vi "calculator.vi"() -> ()   [LabVIEW 2019]
doc: "Use this template to build a producer/consumer design pattern with events to produce queue items. Use this design pattern instead of the User Interface Event Handler pattern for user interfaces when you want to execute code asynchronously in response to an event without slowing the user interface responsiveness."
uses:
  control/command control.ctl
panel:
  in  "Divide":bool
  in  "Multiply":bool
  out "Array 2":string[](array[string])
  out "Array":dbl[](array[numeric])
  in  "Minus":bool
  in  "Equal":bool
  in  "Add":bool
  in  "Off":bool
  out "error out":errorcluster
  in  "Decimal Point":bool
  in  "Button 9":bool
  in  "Button 8":bool
  in  "Button 7":bool
  in  "Button 6":bool
  in  "Button 5":bool
  in  "Button 4":bool
  in  "Button 3":bool
  out "Screen":string
  in  "Button 2":bool
  in  "Button 1":bool
  in  "Button 0":bool
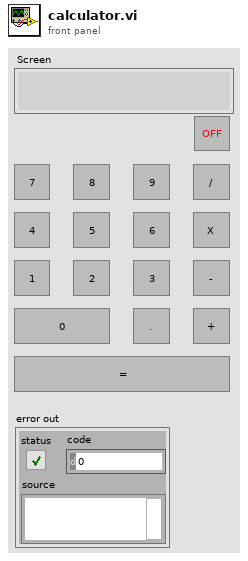
[diagram p1: front panel]
types:
  T1 = typedef "command control.ctl" = enum16{"Multiply", "Divide", "Initialize", "Minus", "Equal", "Add", "Decimal Point", "Number"}
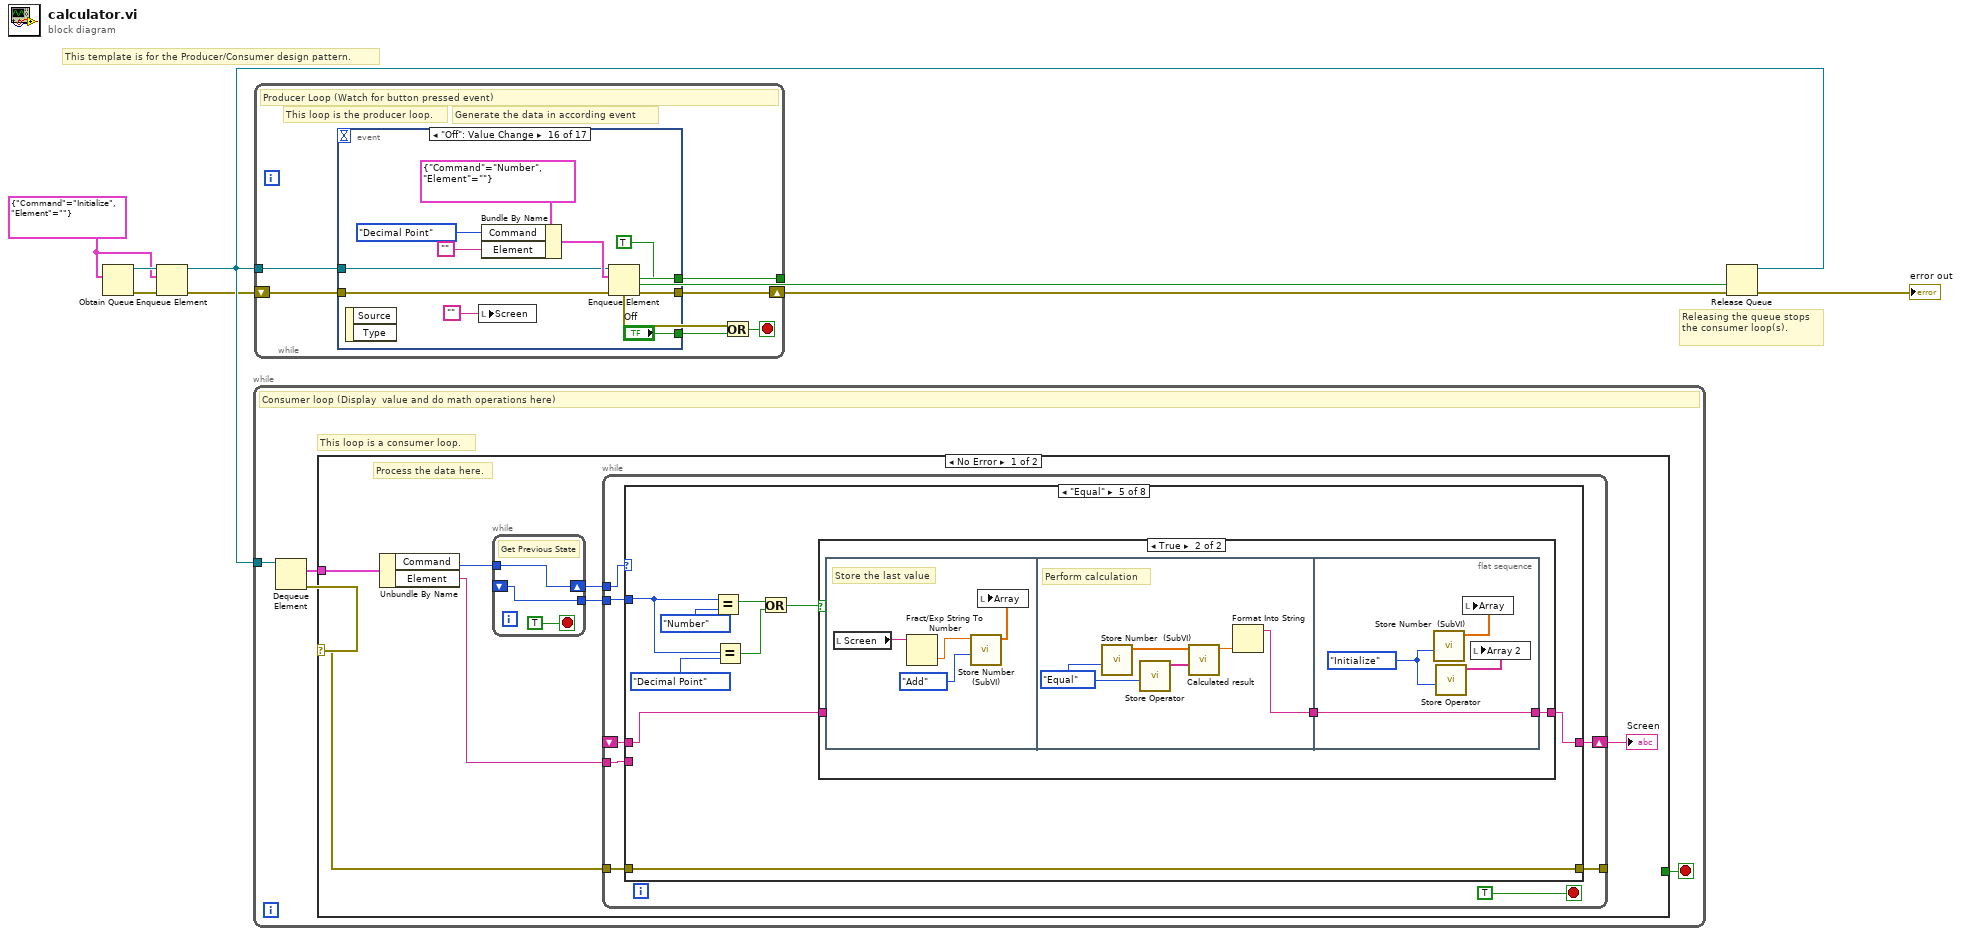
[diagram p0: block diagram]
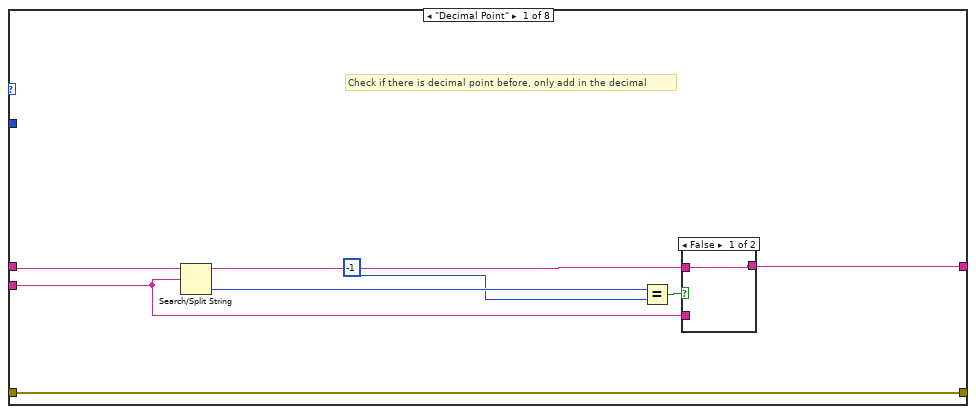
[diagram p2: hidden frame]
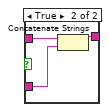
[diagram p3: hidden frame]
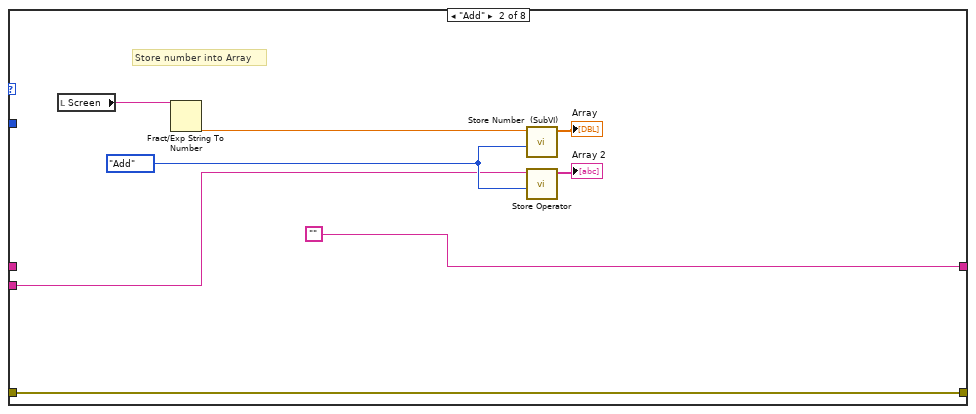
[diagram p4: hidden frame]
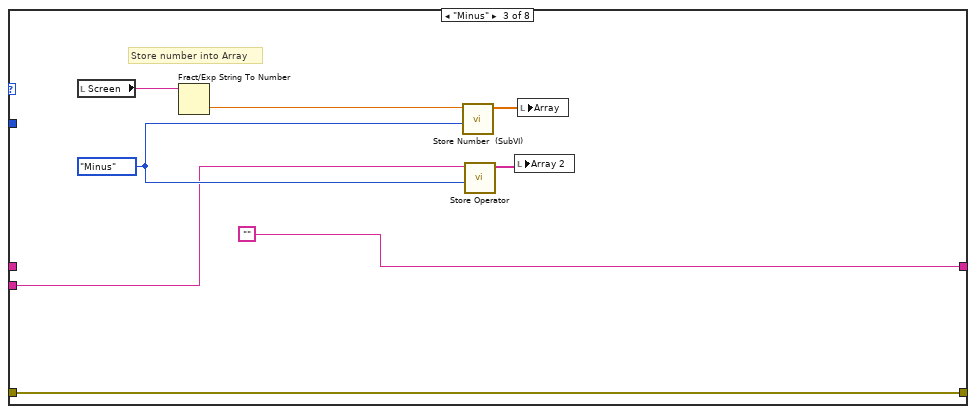
[diagram p5: hidden frame]
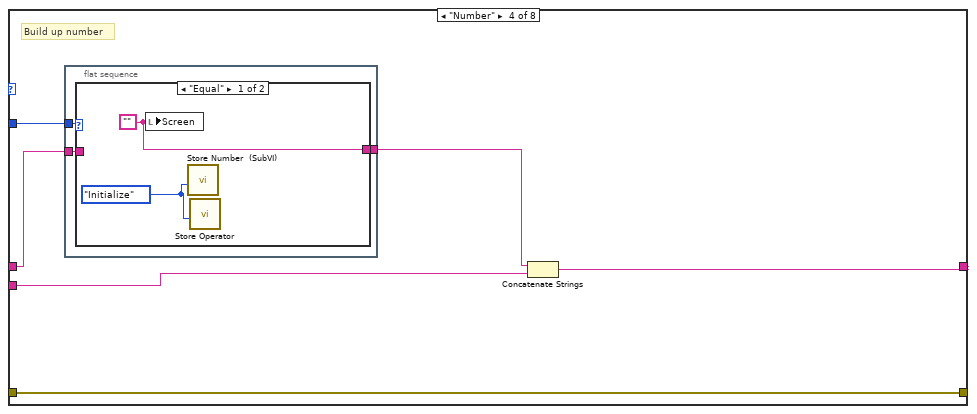
[diagram p6: hidden frame]
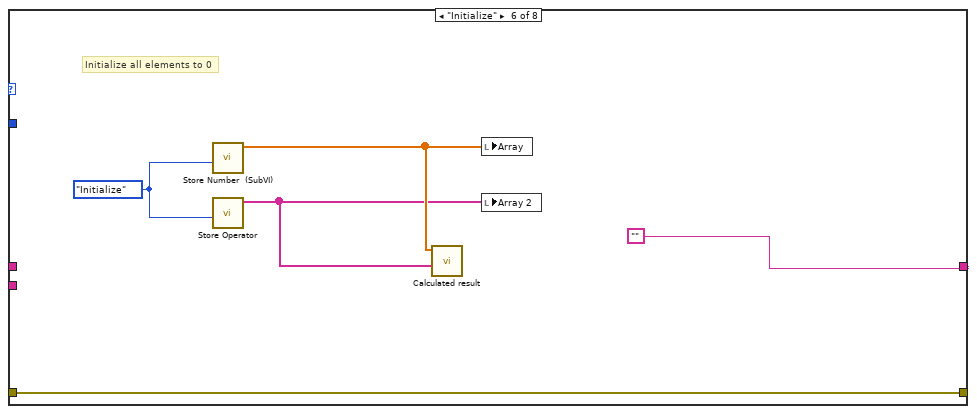
[diagram p9: hidden frame]
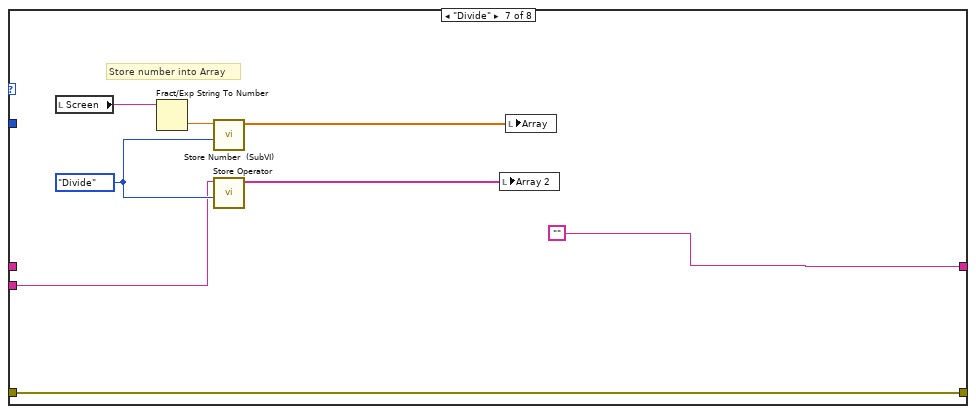
[diagram p10: hidden frame]
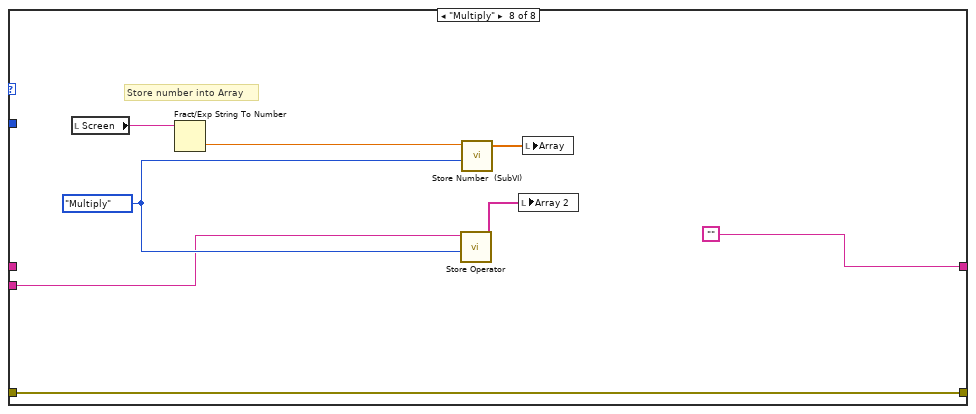
[diagram p11: hidden frame]
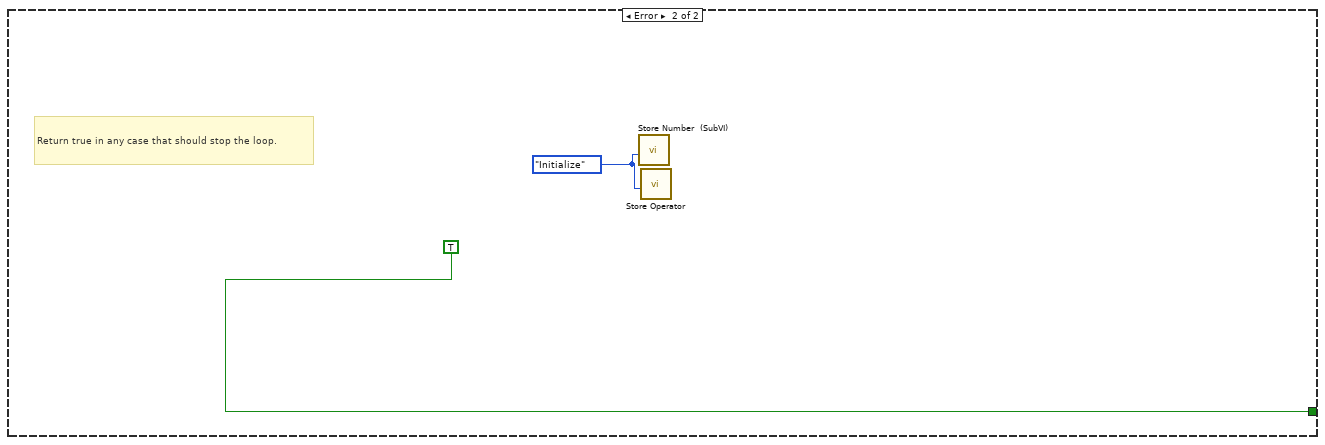
[diagram p12: hidden frame]
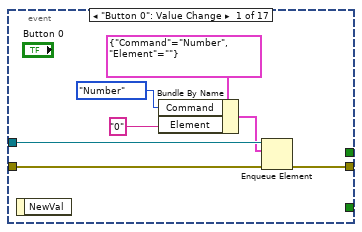
[diagram p13: hidden frame]
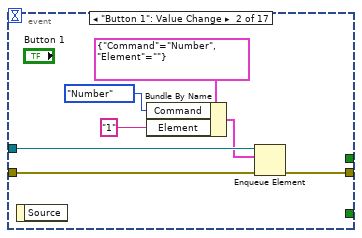
[diagram p14: hidden frame]
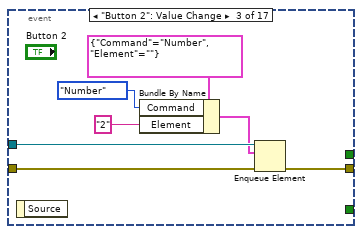
[diagram p15: hidden frame]
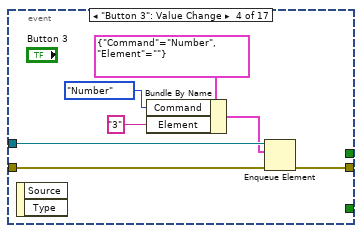
[diagram p16: hidden frame]
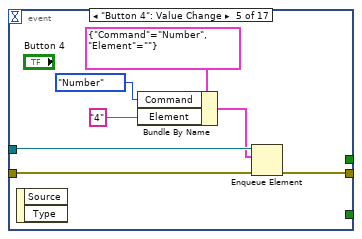
[diagram p17: hidden frame]
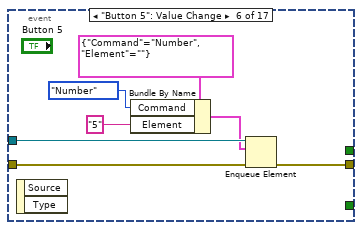
[diagram p18: hidden frame]
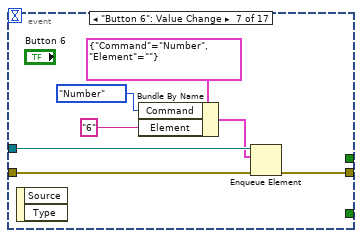
[diagram p19: hidden frame]
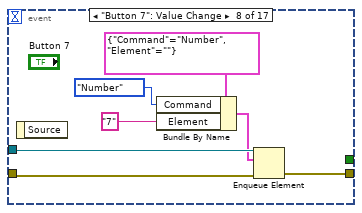
[diagram p20: hidden frame]
diagram:
  w1 = cluster{"Command":T1, "Element":string} {"Command"=enum."Initialize", "Element"=""} ("input cluster")
  # "Releasing the queue stops the consumer loop(s)."
  # "This template is for the Producer/Consumer design pattern."
  n1 = Obtain Queue(element data type=w1) -> (queue out=w7:refnum<queue>, error out=w3:errorcluster)  [unwired: 4 in, 1 out]
  n2 = Enqueue Element(queue=w7, element=w1, error in (no error)=w3) -> (queue out=w4:refnum<queue>, error out=w2:errorcluster)  [unwired: 1 in, 1 out]
  n3 = while {
    tunnel: w4 -> [w12]
    stop <- w10 stop-if-true
    # "This loop is a consumer loop."
    # "Consumer loop (Display  value and do math operations here)"
    n4 = Dequeue Element(queue=w12) -> (element=w9:cluster{"Command":T1, "Element":string}, error out=w11:errorcluster)  [unwired: 2 in, 2 out]
    n5 = case shown="No Error" w11 {
      selector: w11 -> [w16 _]
      tunnel: [_ TRUE] -> w10
      tunnel: w9 -> [w19 _]
      frame No Error {
        # "Process the data here."
        n6 = Unbundle By Name(w19) -> ("Command"=w17:T1, "Element"=w18:string)
        n7 = while {
          shift-right: [w115] -> w15
          shift-left: _ -> [w114]
          tunnel: w17 -> [w115]
          tunnel: [w114] -> w14
          stop <- TRUE stop-if-true
          # "Get Previous State"
        }
        n8 = while {
          shift-right: [w21] -> w13
          shift-left: _ -> [w26]
          tunnel: w18 -> [w25]
          tunnel: w15 -> [w24]
          tunnel: w16 -> [w23]
          tunnel: [w22] -> _
          tunnel: w14 -> [w20]
          stop <- TRUE stop-if-true
          n9 = case shown="\"Equal\"" w24 {
            tunnel: w26 -> [w32 _ _ w56 w68 _ _ _]
            tunnel: [w28 "" "" w59 w75 "" "" ""] -> w21
            tunnel: w25 -> [w31 w40 w48 w61 _ _ w98 w111]
            tunnel: w23 -> [w29 w47 w55 w60 w76 w97 w101 w108]
            tunnel: [w29 w47 w55 w60 w76 w97 w101 w108] -> w22
            tunnel: w20 -> [_ _ _ w58 w69 _ _ _]
            frame "Decimal Point" {
              # "Check if there is decimal point before, only add in the decimal"
              n10 = Search/Split String(string=w32, search string/char (-)=w31) -> (substring before match=w30:string, offset of match=w35:i32)  [unwired: 1 in, 1 out]
              n11 = Equal?(x=w35, y=-1) -> (x = y?=w33:bool)
              n12 = case shown="False" w33 {
                tunnel: w31 -> [_ w39]
                tunnel: [w36 w38] -> w28
                tunnel: w30 -> [w36 w37]
                frame False {
                }
                frame True {
                  n13 = Concatenate Strings(w37, w39) -> (w38:string)
                }
              }
            }
            frame "Add" {
              w43 = command_control."Add" ("Command")
              # "Store number into Array"
              n14 = local read "Screen"() -> (w45:string)
              n15 = Fract/Exp String To Number(string=w45) -> (number=w44:dbl)  [unwired: 3 in, 1 out]
              n16 = call "Store Number  (SubVI).vi"("Command"=w43, "Numeric"=w44) -> ("Array"=→"Array":dbl[])  [unwired: 9 in]
              n17 = call "Store Operator.vi"("Command"=w43, "String"=w40) -> ("Array"=→"Array 2":string[])  [unwired: 9 in]
            }
            frame "Minus" {
              w51 = command_control."Minus" ("Command")
              # "Store number into Array"
              n18 = local read "Screen"() -> (w53:string)
              n19 = Fract/Exp String To Number(string=w53) -> (number=w52:dbl)  [unwired: 3 in, 1 out]
              n20 = call "Store Number  (SubVI).vi"("Command"=w51, "Numeric"=w52) -> ("Array"=w50:dbl[])  [unwired: 9 in]
              n21 = call "Store Operator.vi"("Command"=w51, "String"=w48) -> ("Array"=w49:string[])  [unwired: 9 in]
              n22 = local write "Array 2"(w49) -> ()
              n23 = local write "Array"(w50) -> ()
            }
            frame "Number" {
              # "Build up number"
              n24 = flat-sequence {
                tunnel: w58 -> [w64]
                tunnel: [w63] -> w57
                tunnel: w56 -> [w62]
                frame #0 {
                  n25 = case shown="\"Equal\"" w64 {
                    tunnel: [w66 w67] -> w63
                    tunnel: w62 -> [_ w67]
                    frame "Equal" {
                      w65 = command_control."Initialize" ("Command")
                      w66 = ""
                      n26 = local write "Screen"(w66) -> ()
                      n27 = call "Store Number  (SubVI).vi"("Command"=w65) -> ()  [unwired: 10 in, 1 out]
                      n28 = call "Store Operator.vi"("Command"=w65) -> ()  [unwired: 10 in, 1 out]
                    }
                    frame Default {
                    }
                  }
                }
              }
              n29 = Concatenate Strings(w57, w61) -> (w59:string)
            }
            frame "Equal" {
              n30 = Equal?(x=w69, y=command_control."Number" ("Command")) -> (x = y?=w73:bool)
              n31 = Equal?(x=w69, y=command_control."Decimal Point" ("Command")) -> (x = y?=w71:bool)
              n32 = Or(x=w73, y=w71) -> (x .or. y?=w74:bool)
              n33 = case shown="True" w74 {
                tunnel: [w77 w79] -> w75
                tunnel: w68 -> [w77 _]
                frame False {
                }
                frame True {
                  n34 = flat-sequence {
                    tunnel: [w85] -> w78
                    tunnel: [w91] -> w79
                    tunnel: w78 -> [w91]
                    frame #0 {
                      # "Store the last value"
                      n35 = local read "Screen"() -> (w83:string)
                      n36 = Fract/Exp String To Number(string=w83) -> (number=w82:dbl)  [unwired: 3 in, 1 out]
                      n37 = call "Store Number  (SubVI).vi"("Command"=command_control."Add", "Numeric"=w82) -> ("Array"=w80:dbl[])  [unwired: 9 in]
                      n38 = local write "Array"(w80) -> ()
                    }
                    frame #1 {
                      w84 = command_control."Equal" ("Command")
                      # "Perform calculation"
                      n39 = call "Store Number  (SubVI).vi"("Command"=w84) -> ("Array"=w87:dbl[])  [unwired: 10 in]
                      n40 = call "Store Operator.vi"("Command"=w84) -> ("Array"=w86:string[])  [unwired: 10 in]
                      n41 = call "Calculated result.vi"("Operator Array"=w86, "Number Array"=w87) -> ("Result"=w88:dbl)  [unwired: 9 in]
                      n42 = Format Into String(w88) -> (resulting string=w85:string)  [unwired: 3 in, 1 out]
                    }
                    frame #2 {
                      w92 = command_control."Initialize" ("Command")
                      n43 = call "Store Number  (SubVI).vi"("Command"=w92) -> ("Array"=w90:dbl[])  [unwired: 10 in]
                      n44 = call "Store Operator.vi"("Command"=w92) -> ("Array"=w89:string[])  [unwired: 10 in]
                      n45 = local write "Array"(w90) -> ()
                      n46 = local write "Array 2"(w89) -> ()
                    }
                  }
                }
              }
            }
            frame "Initialize" {
              w93 = command_control."Initialize" ("Command")
              # "Initialize all elements to 0"
              n47 = call "Store Number  (SubVI).vi"("Command"=w93) -> ("Array"=w95:dbl[])  [unwired: 10 in]
              n48 = call "Store Operator.vi"("Command"=w93) -> ("Array"=w94:string[])  [unwired: 10 in]
              n49 = call "Calculated result.vi"("Operator Array"=w94, "Number Array"=w95) -> ()  [unwired: 9 in, 1 out]
              n50 = local write "Array"(w95) -> ()
              n51 = local write "Array 2"(w94) -> ()
            }
            frame "Divide" {
              w104 = command_control."Divide" ("Command")
              # "Store number into Array"
              n52 = local read "Screen"() -> (w103:string)
              n53 = Fract/Exp String To Number(string=w103) -> (number=w105:dbl)  [unwired: 3 in, 1 out]
              n54 = call "Store Number  (SubVI).vi"("Command"=w104, "Numeric"=w105) -> ("Array"=w100:dbl[])  [unwired: 9 in]
              n55 = call "Store Operator.vi"("Command"=w104, "String"=w98) -> ("Array"=w99:string[])  [unwired: 9 in]
              n56 = local write "Array 2"(w99) -> ()
              n57 = local write "Array"(w100) -> ()
            }
            frame "Multiply" {
              w112 = command_control."Multiply" ("Command")
              # "Store number into Array"
              n58 = local read "Screen"() -> (w110:string)
              n59 = Fract/Exp String To Number(string=w110) -> (number=w113:dbl)  [unwired: 3 in, 1 out]
              n60 = call "Store Operator.vi"("Command"=w112, "String"=w111) -> ("Array"=w106:string[])  [unwired: 9 in]
              n61 = call "Store Number  (SubVI).vi"("Command"=w112, "Numeric"=w113) -> ("Array"=w107:dbl[])  [unwired: 9 in]
              n62 = local write "Array 2"(w106) -> ()
              n63 = local write "Array"(w107) -> ()
            }
          }
        }
        "Screen" <- w13
      }
      frame Error {
        w117 = command_control."Initialize" ("Command")
        # "Return true in any case that should stop the loop."
        n64 = call "Store Number  (SubVI).vi"("Command"=w117) -> ()  [unwired: 10 in, 1 out]
        n65 = call "Store Operator.vi"("Command"=w117) -> ()  [unwired: 10 in, 1 out]
      }
    }
  }
  n66 = while {
    shift-right: [w120] -> w8
    shift-left: w2 -> [w123]
    tunnel: w4 -> [w124]
    tunnel: [w119] -> w5
    stop <- w121 stop-if-true
    # "Generate the data in according event"
    # "This loop is the producer loop."
    # "Producer Loop (Watch for button pressed event)"
    n67 = event shown="[15] \"Off\": Value Change" {
      selector: _ -> [_ _ _ _ _ _ _ _ _ _ _ _ _ _ _ _ _]
      dyn-events: _ -> [_ _ _ _ _ _ _ _ _ _ _ _ _ _ _ _ _]
      timeout: _ -> [_ _ _ _ _ _ _ _ _ _ _ _ _ _ _ _ _]
      tunnel: w124 -> [w131 w138 w145 w150 w157 w164 w171 w178 w185 w192 w199 w206 w213 w220 w227 w233 w243]
      tunnel: w123 -> [w130 w137 w144 w151 w158 w165 w172 w179 w186 w193 w200 w207 w214 w221 w228 w238 w244]
      tunnel: [w129 w136 w143 w152 w159 w166 w173 w180 w187 w194 w201 w208 w215 w222 w229 w239 w245] -> w120
      tunnel: [_ _ _ _ _ _ _ _ _ _ _ _ _ _ _ "Off" _] -> w122
      tunnel: [_ _ _ _ _ _ _ _ _ _ _ _ _ _ _ TRUE _] -> w119
      event "Button 0": Value Change {
        n68 = event-data() -> ()  [unwired: 1 in, 1 out]
        n69 = Bundle By Name(cluster=cluster{"Command":T1, "Element":string} {"Command"=enum."Number", "Element"=""} ("input cluster"), "Command"=command_control."Number", "Element"="0" ("element")) -> (w125:cluster{"Command":T1, "Element":string})
        n70 = Enqueue Element(queue=w131, element=w125, error in (no error)=w130) -> (error out=w129:errorcluster)  [unwired: 1 in, 2 out]
      }
      event "Button 1": Value Change {
        n71 = event-data() -> ()  [unwired: 1 in, 1 out]
        n72 = Bundle By Name(cluster=cluster{"Command":T1, "Element":string} {"Command"=enum."Number", "Element"=""} ("input cluster"), "Command"=command_control."Number", "Element"="1" ("element")) -> (w135:cluster{"Command":T1, "Element":string})
        n73 = Enqueue Element(queue=w138, element=w135, error in (no error)=w137) -> (error out=w136:errorcluster)  [unwired: 1 in, 2 out]
      }
      event "Button 2": Value Change {
        n74 = event-data() -> ()  [unwired: 1 in, 1 out]
        n75 = Bundle By Name(cluster=cluster{"Command":T1, "Element":string} {"Command"=enum."Number", "Element"=""} ("input cluster"), "Command"=command_control."Number", "Element"="2" ("element")) -> (w141:cluster{"Command":T1, "Element":string})
        n76 = Enqueue Element(queue=w145, element=w141, error in (no error)=w144) -> (error out=w143:errorcluster)  [unwired: 1 in, 2 out]
      }
      event "Button 3": Value Change {
        n77 = event-data() -> ()  [unwired: 1 in, 2 out]
        n78 = Bundle By Name(cluster=cluster{"Command":T1, "Element":string} {"Command"=enum."Number", "Element"=""} ("input cluster"), "Command"=command_control."Number", "Element"="3" ("element")) -> (w149:cluster{"Command":T1, "Element":string})
        n79 = Enqueue Element(queue=w150, element=w149, error in (no error)=w151) -> (error out=w152:errorcluster)  [unwired: 1 in, 2 out]
      }
      event "Button 4": Value Change {
        n80 = event-data() -> ()  [unwired: 1 in, 2 out]
        n81 = Bundle By Name(cluster=cluster{"Command":T1, "Element":string} {"Command"=enum."Number", "Element"=""} ("input cluster"), "Command"=command_control."Number", "Element"="4" ("element")) -> (w153:cluster{"Command":T1, "Element":string})
        n82 = Enqueue Element(queue=w157, element=w153, error in (no error)=w158) -> (error out=w159:errorcluster)  [unwired: 1 in, 2 out]
      }
      event "Button 5": Value Change {
        n83 = event-data() -> ()  [unwired: 1 in, 2 out]
        n84 = Bundle By Name(cluster=cluster{"Command":T1, "Element":string} {"Command"=enum."Number", "Element"=""} ("input cluster"), "Command"=command_control."Number", "Element"="5" ("element")) -> (w160:cluster{"Command":T1, "Element":string})
        n85 = Enqueue Element(queue=w164, element=w160, error in (no error)=w165) -> (error out=w166:errorcluster)  [unwired: 1 in, 2 out]
      }
      event "Button 6": Value Change {
        n86 = event-data() -> ()  [unwired: 1 in, 2 out]
        n87 = Bundle By Name(cluster=cluster{"Command":T1, "Element":string} {"Command"=enum."Number", "Element"=""} ("input cluster"), "Command"=command_control."Number", "Element"="6" ("element")) -> (w167:cluster{"Command":T1, "Element":string})
        n88 = Enqueue Element(queue=w171, element=w167, error in (no error)=w172) -> (error out=w173:errorcluster)  [unwired: 1 in, 2 out]
      }
      event "Button 7": Value Change {
        n89 = event-data() -> ()  [unwired: 1 in, 1 out]
        n90 = Bundle By Name(cluster=cluster{"Command":T1, "Element":string} {"Command"=enum."Number", "Element"=""} ("input cluster"), "Command"=command_control."Number", "Element"="7" ("element")) -> (w174:cluster{"Command":T1, "Element":string})
        n91 = Enqueue Element(queue=w178, element=w174, error in (no error)=w179) -> (error out=w180:errorcluster)  [unwired: 1 in, 2 out]
      }
      event "Button 8": Value Change {
        n92 = event-data() -> ()  [unwired: 1 in, 2 out]
        n93 = Bundle By Name(cluster=cluster{"Command":T1, "Element":string} {"Command"=enum."Number", "Element"=""} ("input cluster"), "Command"=command_control."Number", "Element"="8" ("element")) -> (w181:cluster{"Command":T1, "Element":string})
        n94 = Enqueue Element(queue=w185, element=w181, error in (no error)=w186) -> (error out=w187:errorcluster)  [unwired: 1 in, 2 out]
      }
      event "Button 9": Value Change {
        n95 = event-data() -> ()  [unwired: 1 in, 2 out]
        n96 = Bundle By Name(cluster=cluster{"Command":T1, "Element":string} {"Command"=enum."Number", "Element"=""} ("input cluster"), "Command"=command_control."Number", "Element"="9" ("element")) -> (w188:cluster{"Command":T1, "Element":string})
        n97 = Enqueue Element(queue=w192, element=w188, error in (no error)=w193) -> (error out=w194:errorcluster)  [unwired: 1 in, 2 out]
      }
      event "Decimal Point": Value Change {
        n98 = event-data() -> ()  [unwired: 1 in, 2 out]
        n99 = Bundle By Name(cluster=cluster{"Command":T1, "Element":string} {"Command"=enum."Number", "Element"=""} ("input cluster"), "Command"=command_control."Decimal Point", "Element"="." ("element")) -> (w197:cluster{"Command":T1, "Element":string})
        n100 = Enqueue Element(queue=w199, element=w197, error in (no error)=w200) -> (error out=w201:errorcluster)  [unwired: 1 in, 2 out]
      }
      event "Add": Value Change {
        n101 = event-data() -> ()  [unwired: 1 in, 1 out]
        n102 = Bundle By Name(cluster=cluster{"Command":T1, "Element":string} {"Command"=enum."Number", "Element"=""} ("input cluster"), "Command"=command_control."Add", "Element"="+" ("element")) -> (w204:cluster{"Command":T1, "Element":string})
        n103 = Enqueue Element(queue=w206, element=w204, error in (no error)=w207) -> (error out=w208:errorcluster)  [unwired: 1 in, 2 out]
      }
      event "Minus": Value Change {
        n104 = event-data() -> ()  [unwired: 1 in, 1 out]
        n105 = Bundle By Name(cluster=cluster{"Command":T1, "Element":string} {"Command"=enum."Number", "Element"=""} ("input cluster"), "Command"=command_control."Minus", "Element"="-" ("element")) -> (w211:cluster{"Command":T1, "Element":string})
        n106 = Enqueue Element(queue=w213, element=w211, error in (no error)=w214) -> (error out=w215:errorcluster)  [unwired: 1 in, 2 out]
      }
      event "Divide": Value Change {
        n107 = event-data() -> ()  [unwired: 1 in, 1 out]
        n108 = Bundle By Name(cluster=cluster{"Command":T1, "Element":string} {"Command"=enum."Number", "Element"=""} ("input cluster"), "Command"=command_control."Divide", "Element"="/" ("element")) -> (w218:cluster{"Command":T1, "Element":string})
        n109 = Enqueue Element(queue=w220, element=w218, error in (no error)=w221) -> (error out=w222:errorcluster)  [unwired: 1 in, 2 out]
      }
      event "Multiply": Value Change {
        n110 = event-data() -> ()  [unwired: 1 in, 1 out]
        n111 = Bundle By Name(cluster=cluster{"Command":T1, "Element":string} {"Command"=enum."Number", "Element"=""} ("input cluster"), "Command"=command_control."Multiply", "Element"="*" ("element")) -> (w225:cluster{"Command":T1, "Element":string})
        n112 = Enqueue Element(queue=w227, element=w225, error in (no error)=w228) -> (error out=w229:errorcluster)  [unwired: 1 in, 2 out]
      }
      event "Off": Value Change {
        n113 = event-data() -> ()  [unwired: 1 in, 2 out]
        n114 = local write "Screen"("") -> ()
        n115 = Bundle By Name(cluster=cluster{"Command":T1, "Element":string} {"Command"=enum."Number", "Element"=""} ("input cluster"), "Command"=command_control."Decimal Point", "Element"="") -> (w234:cluster{"Command":T1, "Element":string})
        n116 = Enqueue Element(queue=w233, element=w234, error in (no error)=w238) -> (error out=w239:errorcluster)  [unwired: 1 in, 2 out]
      }
      event "Equal": Value Change {
        n117 = event-data() -> ()  [unwired: 1 in, 2 out]
        n118 = Bundle By Name(cluster=cluster{"Command":T1, "Element":string} {"Command"=enum."Number", "Element"=""} ("input cluster"), "Command"=command_control."Equal", "Element"="=") -> (w240:cluster{"Command":T1, "Element":string})
        n119 = Enqueue Element(queue=w243, element=w240, error in (no error)=w244) -> (error out=w245:errorcluster)  [unwired: 1 in, 2 out]
      }
    }
    n120 = Or(x=w120, y=w122) -> (x .or. y?=w121:bool)
  }
  n121 = Release Queue(queue=w4, force destroy? (F)=w5, error in (no error)=w8) -> (error out=→"error out":errorcluster)  [unwired: 2 out]
